vi "Eval X-Y(a,t).vi"(4 "number of points":u32=10, 5 "Formulas":string[](array[string])=["", ""], 6 "Parameters":cluster{"name":string, "value":dbl}[](array[cluster]) {"value" format="%.2f"}, 7 "end":dbl=1.0 format="%.2f", 8 "start":dbl format="%.2f") -> (0 "error":i32, 1 "ticks":u32, 2 "Y":dbl[](array[numeric]) format="%.2f", 3 "X":dbl[](array[numeric]) format="%.2f")   [LabVIEW 2020, in "NI_Gmath.lvlib"]
doc: "Calculates the (x, y) coordinates of a curve by calculating the parametric function values of x = f(t) and y = g(t), where t runs over an interval."
uses:
  <vilib>/gmath/NI_Gmath.lvlib
panel:
  # "Example:\n\n number of points: 100 \n start: 0.0\n end: 1.0\n Parameters: (a,1) and (b,2) \n Formulas: sin(t*a)+b and exp(t-a)"
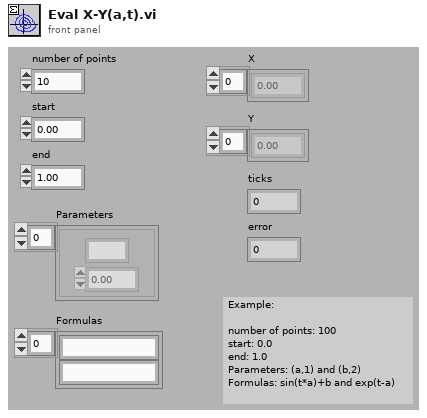
[diagram p1: front panel]
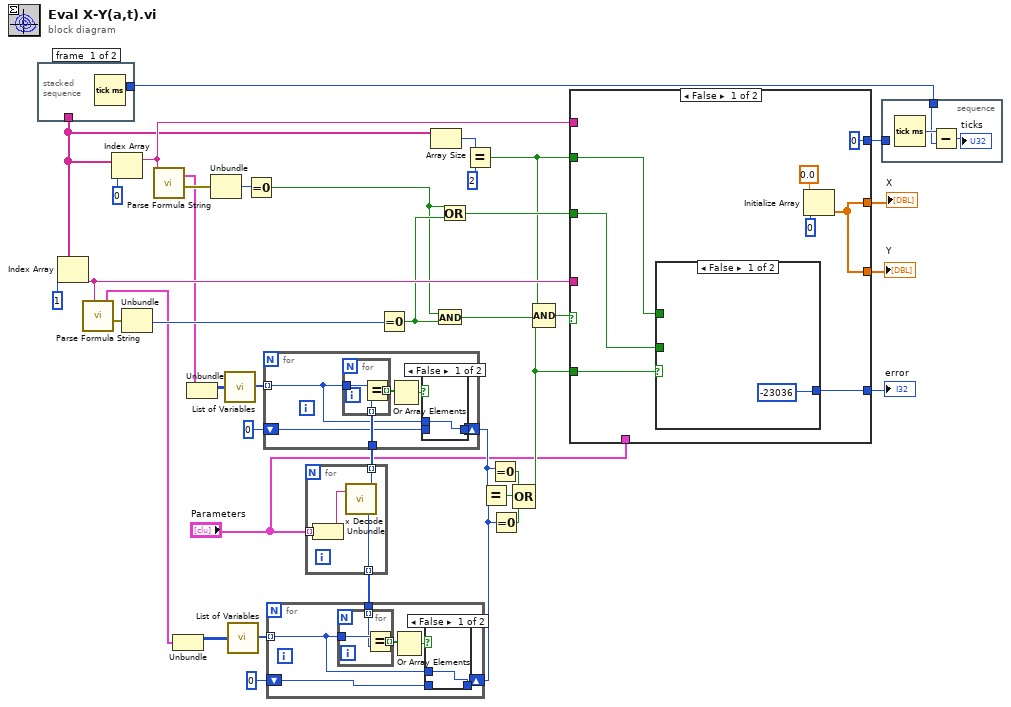
[diagram p0: block diagram]
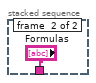
[diagram p4: hidden frame]
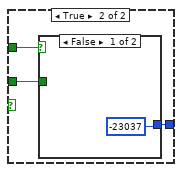
[diagram p5: hidden frame]
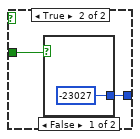
[diagram p6: hidden frame]
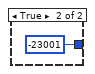
[diagram p7: hidden frame]
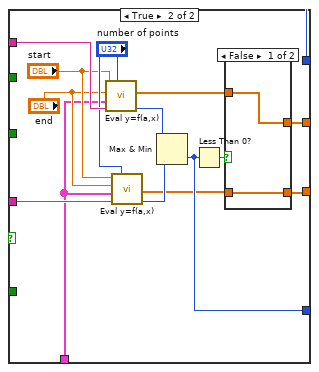
[diagram p8: hidden frame]
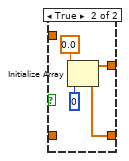
[diagram p9: hidden frame]
diagram:
  n1 = stacked-sequence {
    tunnel: [w40 _] -> w39
    tunnel: [_ "Formulas"] -> w3
    frame #0 {
      n2 = Tick Count (ms)() -> (millisecond timer value=w40:u32)
    }
    frame #1 {
    }
  }
  n3 = Index Array(array=w3, index=1) -> (element=w24:string)
  n4 = call <vilib>:"Parse Formula String.vi"("formula"=w24) -> ("error out"=w30:errorcluster, "Parsed Formula"=w14:cluster{"Table":i32[][], "Y Values":dbl[]})  [unwired: 1 in]
  n5 = Index Array(array=w3, index=0) -> (element=w25:string)
  n6 = Unbundle(w30) -> ("code"=w31:i32)  [unwired: 2 out]
  n7 = call <vilib>:"Parse Formula String.vi"("formula"=w25) -> ("error out"=w35:errorcluster, "Parsed Formula"=w20:cluster{"Table":i32[][], "Y Values":dbl[]})  [unwired: 1 in]
  n8 = Unbundle(w14) -> ("Table"=w16:i32[][])  [unwired: 1 out]
  n9 = Unbundle(w20) -> ("Table"=w21:i32[][])  [unwired: 1 out]
  n10 = Unbundle(w35) -> ("code"=w34:i32)  [unwired: 2 out]
  n11 = call <vilib>:"List of Variables.vi"("Table"=w21) -> ("List of variables"=w19:i32[])
  n12 = call <vilib>:"List of Variables.vi"("Table"=w16) -> ("List of variables"=w17:i32[])
  n13 = Equal To 0?(x=w34) -> (x = 0?=w2:bool)
  n14 = for {
    tunnel: "Parameters" -> [w44] mode=indexing
    tunnel: [w42] -> w18 mode=indexing
    tunnel: [w42] -> w13 mode=indexing
    n15 = Unbundle(w44) -> ("name"=w43:string)  [unwired: 1 out]
    n16 = call <vilib>:"x Decode.vi"("x string"=w43) -> ("number"=w42:i32)  [unwired: 1 in, 1 out]
  }
  n17 = for {
    tunnel: w18 -> [w50]
    shift-right: [w46] -> w9
    shift-left: 0 -> [w47]
    tunnel: w19 -> [w45] mode=indexing
    n18 = for {
      tunnel: w50 -> [w53] mode=indexing
      tunnel: w45 -> [w55]
      tunnel: [w54] -> w49 mode=indexing
      n19 = Equal?(x=w55, y=w53) -> (x = y?=w54:bool)
    }
    n20 = Or Array Elements(Boolean array=w49) -> (logical OR=w48:bool)
    n21 = case shown="False" w48 {
      tunnel: w47 -> [_ w52]
      tunnel: [w51 w52] -> w46
      tunnel: w45 -> [w51 _]
      frame False {
      }
      frame True {
      }
    }
  }
  n22 = for {
    shift-right: [w58] -> w6
    shift-left: 0 -> [w59]
    tunnel: w17 -> [w57] mode=indexing
    tunnel: w13 -> [w56]
    n23 = for {
      tunnel: w57 -> [w66]
      tunnel: [w65] -> w61 mode=indexing
      tunnel: w56 -> [w64] mode=indexing
      n24 = Equal?(x=w66, y=w64) -> (x = y?=w65:bool)
    }
    n25 = Or Array Elements(Boolean array=w61) -> (logical OR=w60:bool)
    n26 = case shown="False" w60 {
      tunnel: w59 -> [_ w63]
      tunnel: [w62 w63] -> w58
      tunnel: w57 -> [w62 _]
      frame False {
      }
      frame True {
      }
    }
  }
  n27 = Equal To 0?(x=w31) -> (x = 0?=w23:bool)
  n28 = Array Size(array=w3) -> (size(s)=w29:i32)
  n29 = And(x=w2, y=w23) -> (x .and. y?=w10:bool)
  n30 = Or(x=w2, y=w23) -> (x .or. y?=w26:bool)
  n31 = Equal?(x=w29, y=2) -> (x = y?=w11:bool)
  n32 = Equal?(x=w9, y=w6) -> (x = y?=w7:bool)
  n33 = Equal To 0?(x=w9) -> (x = 0?=w8:bool)
  n34 = Equal To 0?(x=w6) -> (x = 0?=w5:bool)
  n35 = Compound Arithmetic op=OR(w8, w7, w5) -> (w4:bool)
  n36 = Compound Arithmetic op=AND(w11, w10, w4) -> (w12:bool)
  n37 = case shown="False" w12 {
    tunnel: [w71 w85] -> w38
    tunnel: [w71 w87] -> w37
    tunnel: [0 0] -> w36
    tunnel: [w70 w90] -> w27
    tunnel: w11 -> [w69 _]
    tunnel: w26 -> [w68 _]
    tunnel: w25 -> [_ w97]
    tunnel: w24 -> [_ w93]
    tunnel: "Parameters" -> [_ w84]
    tunnel: w4 -> [w67 _]
    frame False {
      n38 = case shown="False" w67 {
        tunnel: w68 -> [_ w78]
        tunnel: w69 -> [_ w77]
        tunnel: [-23036 w76] -> w70
        frame False {
        }
        frame True {
          n39 = case shown="False" w77 {
            tunnel: w78 -> [_ w81]
            tunnel: [-23037 w80] -> w76
            frame False {
            }
            frame True {
              n40 = case shown="False" w81 {
                tunnel: [-23027 -23001] -> w80
                frame False {
                }
                frame True {
                }
              }
            }
          }
        }
      }
      n41 = Initialize Array(0.0, 0) -> (w71:dbl[])
    }
    frame True {
      n42 = call <vilib>:"Eval y=f(a,x).vi"("number of points"="number of points", "formula"=w97, "Parameters"=w84, "end"="end", "start"="start") -> ("error"=w92:i32, "Y"=w88:dbl[])  [unwired: 2 out]
      n43 = call <vilib>:"Eval y=f(a,x).vi"("number of points"="number of points", "formula"=w93, "Parameters"=w84, "end"="end", "start"="start") -> ("error"=w91:i32, "Y"=w86:dbl[])  [unwired: 2 out]
      n44 = Max & Min(x=w92, y=w91) -> (min(x,y)=w90:i32)  [unwired: 1 out]
      n45 = Less Than 0?(x=w90) -> (x < 0?=w89:bool)
      n46 = case shown="False" w89 {
        tunnel: w88 -> [w100 _]
        tunnel: [w100 w101] -> w87
        tunnel: [w99 w101] -> w85
        tunnel: w86 -> [w99 _]
        frame False {
        }
        frame True {
          n47 = Initialize Array(0.0, 0) -> (w101:dbl[])
        }
      }
    }
  }
  "X" <- w37
  "Y" <- w38
  "error" <- w27
  n48 = stacked-sequence {
    tunnel: w39 -> [w104]
    tunnel: w36 -> [_]
    frame #0 {
      n49 = Tick Count (ms)() -> (millisecond timer value=w105:u32)
      n50 = Subtract(x=w105, y=w104) -> (x-y=→"ticks":u32)
    }
  }
